vi "Update NIC Ctrls.vi"(8 "Error In":errorcluster, 10 "Selected NIC":u16, 11 "Install LV Data":T1={"SSH Session"=refnum, "Status Log"="", "Detailed Log"="", "Credentials"={"Hostname or IP"="192.168.7.2", "Username"="root", "Password"=""}, "Target Info"={"OS Version"="", "CPU"="", "Systemd Version"="", "Internet Access"=FALSE, "Device Type"="", "LV Installed Ver"="", "LV Available Ver"="", "LV Upgrade Available"=FALSE, "Hostname"="", "NIC Info"=[]}, "Reboot Required?"=FALSE}) -> (0 "Error Out":errorcluster, 3 "Install LV Data":T1={"SSH Session"=refnum, "Status Log"="", "Detailed Log"="", "Credentials"={"Hostname or IP"="192.168.7.2", "Username"="root", "Password"=""}, "Target Info"={"OS Version"="", "CPU"="", "Systemd Version"="", "Internet Access"=FALSE, "Device Type"="", "LV Installed Ver"="", "LV Available Ver"="", "LV Upgrade Available"=FALSE, "Hostname"="", "NIC Info"=[]}, "Reboot Required?"=FALSE})   [LabVIEW 2019, in "LMH-LINX.lvlib"]
uses:
  <vilib>/MakerHub/LINX/LMH-LINX.lvlib
  <vilib>/MakerHub/LINX/Private/Utilties/Target Management/Install LV Data.ctl
  <vilib>/MakerHub/LINX/Private/Utilties/Target Management/Target Info.ctl
  <vilib>/MakerHub/LINX/Private/Utilties/Target Management/NIC Info.ctl
  <vilib>/MakerHub/LINX/Private/Utilties/Target Management/NIC Mode.ctl
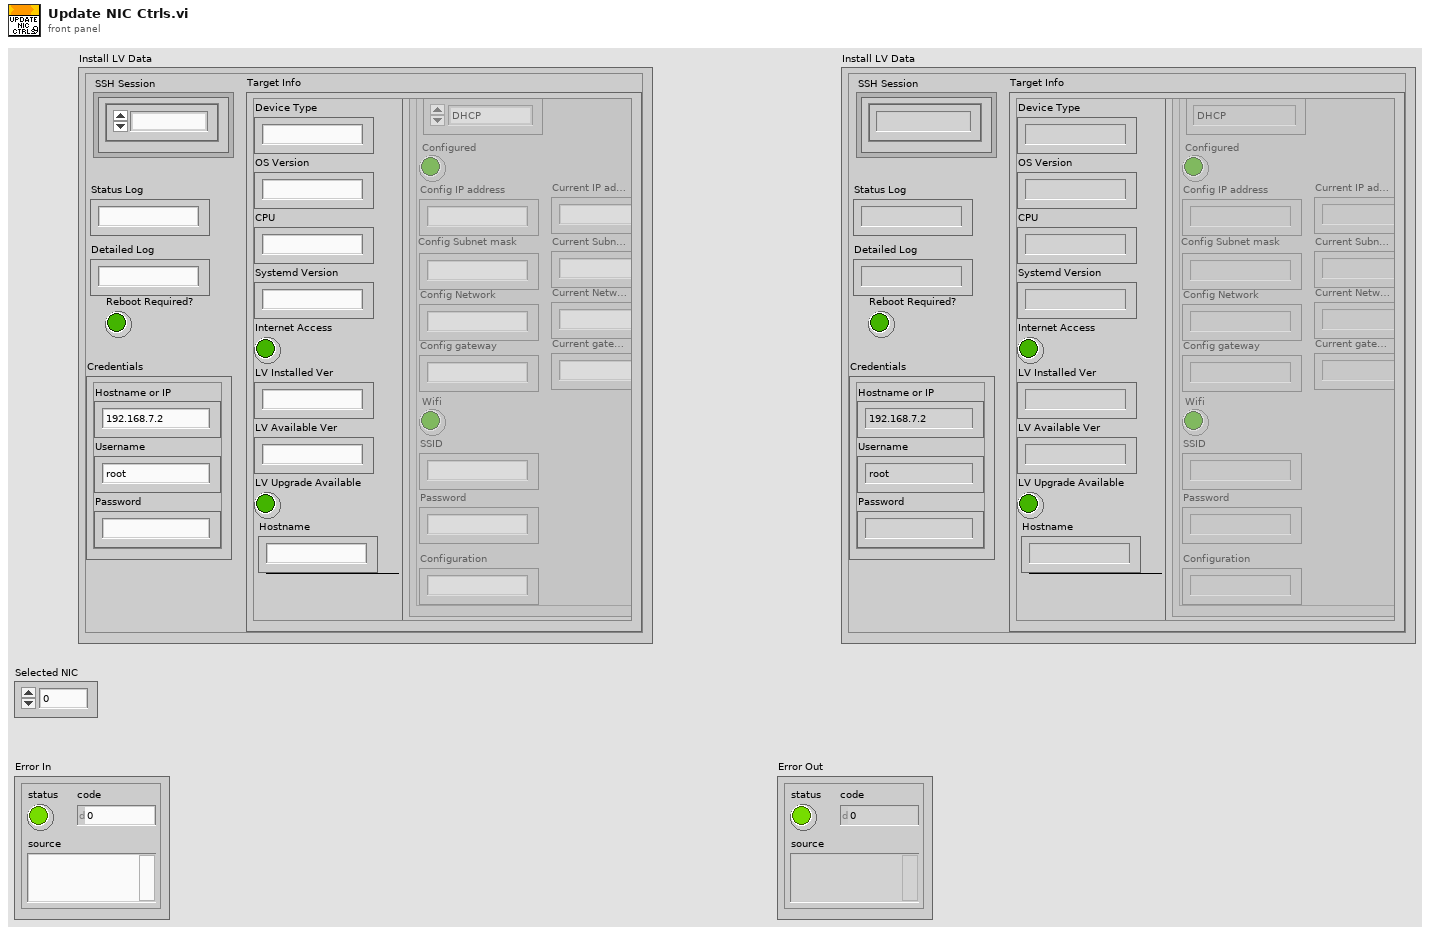
[diagram p1: front panel]
types:
  T1 = typedef "LMH-LINX.lvlib/Install LV Data.ctl" = cluster{"SSH Session":refnum<k1>, "Status Log":string, "Detailed Log":string, "Credentials":cluster{"Hostname or IP":string, "Username":string, "Password":string}, "Target Info":T2, "Reboot Required?":bool}
  T2 = typedef "LMH-LINX.lvlib/Target Info.ctl" = cluster{"OS Version":string, "CPU":string, "Systemd Version":string, "Internet Access":bool, "Device Type":string, "LV Installed Ver":string, "LV Available Ver":string, "LV Upgrade Available":bool, "Hostname":string, "NIC Info":T3[]}
  T3 = typedef "LMH-LINX.lvlib/NIC Info.ctl" = cluster{"Name":string, "NIC Mode":T4, "Configured":bool, "Config IP address":string, "Config Subnet mask":string, "Config Network":string, "Config gateway":string, "Wifi":bool, "SSID":string, "Password":string, "Configuration":string, "Current IP address":string, "Current Subnet mask":string, "Current gateway":string, "Current Network":string}
  T4 = typedef "LMH-LINX.lvlib/NIC Mode.ctl" = enum16{"DHCP", "Static", "Loopback"}
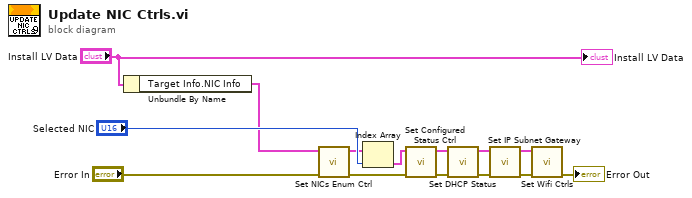
[diagram p0: block diagram]
diagram:
  n1 = Unbundle By Name("Install LV Data") -> ("Target Info.NIC Info"=w2:T3[])
  n2 = call <vilib>:"Set NICs Enum Ctrl.vi"("Error In"="Error In", "NIC Info"=w2) -> ("Error Out"=w6:errorcluster, "NIC Info"=w5:T3[])  [unwired: 8 in]
  n3 = Index Array(array=w5, index="Selected NIC") -> (element=w4:T3)
  n4 = call <vilib>:"Set Configured Status Ctrl.vi"("Error In"=w6, "NIC Info"=w4) -> ("Error Out"=w12:errorcluster, "NIC Info"=w11:T3)  [unwired: 8 in]
  n5 = call <vilib>:"Set DHCP Status.vi"("Error In"=w12, "NIC Info"=w11) -> ("Error Out"=w10:errorcluster, "NIC Info"=w9:T3)  [unwired: 8 in]
  n6 = call <vilib>:"Set IP Subnet Gateway.vi"("Error In"=w10, "NIC Info"=w9) -> ("Error Out"=w8:errorcluster, "NIC Info"=w7:T3)  [unwired: 8 in]
  n7 = call <vilib>:"Set Wifi Ctrls.vi"("Error In"=w8, "NIC Info"=w7) -> ("Error Out"=→"Error Out":errorcluster)  [unwired: 8 in, 1 out]
  "Install LV Data" <- "Install LV Data"
